vi "Update Credit.vi"(8 "error in (no error)":errorcluster, 9 "Change":dbl, 10 "Credit":dbl, 11 "Dinero in":refnum<class "Dinero.lvclass">) -> (0 "error out":errorcluster, 3 "Dinero out":refnum<class "Dinero.lvclass">)   [LabVIEW 2020, in "Dinero.lvlib" / "Dinero.lvclass"]
uses:
  Dinero.lvclass
  Dinero.lvclass/Dinero.ctl
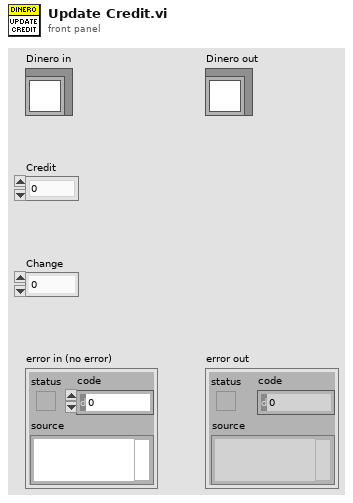
[diagram p1: front panel]
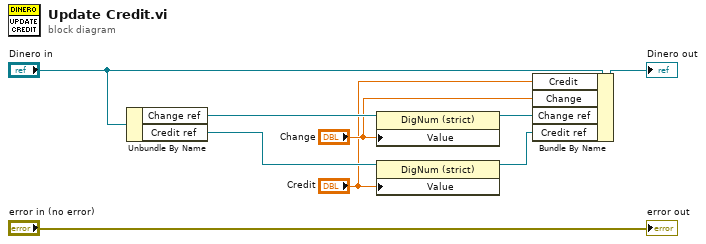
[diagram p0: block diagram]
diagram:
  n1 = Unbundle By Name("Dinero in") -> ("Change ref"=w7:refnum<vi>, "Credit ref"=w6:refnum<vi>)
  n2 = property class="DigNum (strict)"(reference=w7, "Value"="Change") -> (reference out=w4:refnum<vi>)  [unwired: 1 in, 1 out]
  n3 = property class="DigNum (strict)"(reference=w6, "Value"="Credit") -> (reference out=w3:refnum<vi>)  [unwired: 1 in, 1 out]
  n4 = Bundle By Name(cluster="Dinero in", "Credit"="Credit", "Change"="Change", "Change ref"=w4, "Credit ref"=w3) -> (→"Dinero out":refnum<class "Dinero.lvclass">)
  "error out" <- "error in (no error)"
